vi "ClimbWeightQueue.vi"(7 "Action":T1, 8 "error in (no error)":errorcluster, 9 "Swing Out?":bool, 10 "ClimbWeightSol4":T2={"DevStatus"={"status"=FALSE, "code"=0, "source"=""}, "Solenoid Module"=enum."Solenoid Module 1", "Forward Solenoid Channel"=enum."Invalid", "Reverse Solenoid Channel"=enum."Invalid"}, 11 "ClimbWeightSol3":T2={"DevStatus"={"status"=FALSE, "code"=0, "source"=""}, "Solenoid Module"=enum."Solenoid Module 1", "Forward Solenoid Channel"=enum."Invalid", "Reverse Solenoid Channel"=enum."Invalid"}) -> (0 "error out":errorcluster)   [LabVIEW 2013]
uses:
  <vilib>/Rock Robotics/WPI/Solenoid/WPI_SolenoidDevRef.ctl
  <vilib>/Rock Robotics/SystemInterfaces/Typedef/FPGA_TypedefSolenoidModule.ctl
  <vilib>/Rock Robotics/WPI/Solenoid/WPI_SolenoidChannel.ctl
  ActionEnum.ctl
  <vilib>/Rock Robotics/WPI/Solenoid/WPI_SolenoidValue.ctl
  <vilib>/Rock Robotics/WPI/Solenoid/WPI_SolenoidSetEnum.vi
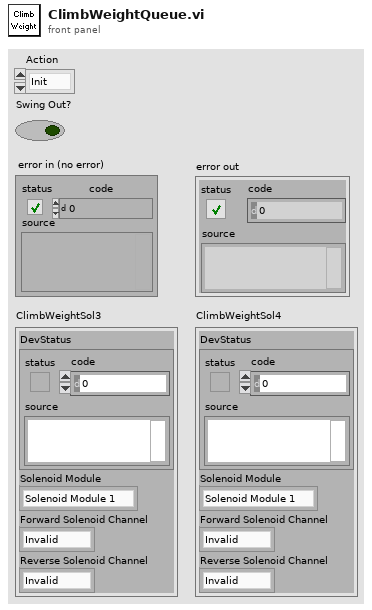
[diagram p1: front panel]
types:
  T1 = typedef "ActionEnum.ctl" = enum16{"Init", "SetValue"}
  T2 = typedef "WPI_SolenoidDevRef.ctl" = cluster{"DevStatus":errorcluster, "Solenoid Module":T3, "Forward Solenoid Channel":T4, "Reverse Solenoid Channel":T4}
  T3 = typedef "FPGA_TypedefSolenoidModule.ctl" = enum16{"Solenoid Module 1", "Solenoid Module 2"}
  T4 = typedef "WPI_SolenoidChannel.ctl" = enum8{"Solenoid 1", "Solenoid 2", "Solenoid 3", "Solenoid 4", "Solenoid 5", "Solenoid 6", "Solenoid 7", "Solenoid 8", "Invalid"}
  T5 = typedef "WPI_SolenoidValue.ctl" = enum16{"Off", "On", "Forward", "Reverse"}
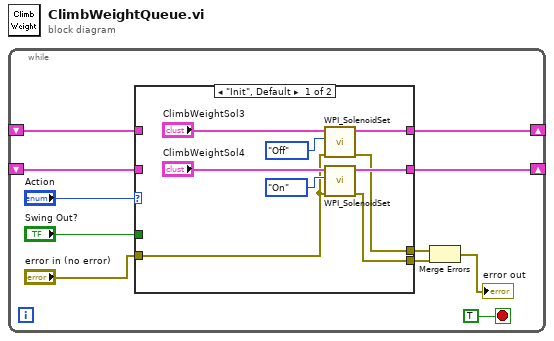
[diagram p0: block diagram]
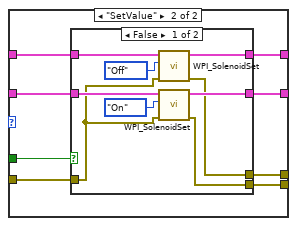
[diagram p2: hidden frame]
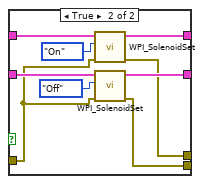
[diagram p3: hidden frame]
diagram:
  n1 = while {
    shift-right: [w6] -> _
    shift-left: _ -> [w10]
    shift-right: [w7] -> _
    shift-left: _ -> [w9]
    stop <- TRUE stop-if-true
    n2 = case shown="\"Init\", Default" "Action" {
      tunnel: [w17 w28] -> w6
      tunnel: [w15 w27] -> w7
      tunnel: w10 -> [_ w24]
      tunnel: w9 -> [_ w23]
      tunnel: "Swing Out?" -> [_ w26]
      tunnel: "error in (no error)" -> [w14 w25]
      tunnel: [w13 w22] -> w3
      tunnel: [w12 w21] -> w2
      frame "Init", Default {
        n3 = call-poly <vilib>:"WPI_SolenoidSet.vi"("error in (no error)"=w14, "Value"=WPI_SolenoidValue."Off", "SolenoidDevRef"="ClimbWeightSol3") -> ("error out"=w13:errorcluster, "SolenoidDevRef"=w17:T2)  [unwired: 7 in]
        n4 = call-poly <vilib>:"WPI_SolenoidSet.vi"("error in (no error)"=w14, "Value"=WPI_SolenoidValue."On", "SolenoidDevRef"="ClimbWeightSol4") -> ("error out"=w12:errorcluster, "SolenoidDevRef"=w15:T2)  [unwired: 7 in]
      }
      frame "SetValue" {
        n5 = case shown="False" w26 {
          tunnel: [w34 w45] -> w27
          tunnel: [w35 w46] -> w28
          tunnel: w25 -> [w31 w40]
          tunnel: w24 -> [w33 w42]
          tunnel: w23 -> [w32 w41]
          tunnel: [w29 w39] -> w21
          tunnel: [w30 w38] -> w22
          frame False {
            n6 = call-poly <vilib>:"WPI_SolenoidSet.vi"("error in (no error)"=w31, "Value"=WPI_SolenoidValue."Off", "SolenoidDevRef"=w33) -> ("error out"=w30:errorcluster, "SolenoidDevRef"=w35:T2)  [unwired: 7 in]
            n7 = call-poly <vilib>:"WPI_SolenoidSet.vi"("error in (no error)"=w31, "Value"=WPI_SolenoidValue."On", "SolenoidDevRef"=w32) -> ("error out"=w29:errorcluster, "SolenoidDevRef"=w34:T2)  [unwired: 7 in]
          }
          frame True {
            n8 = call-poly <vilib>:"WPI_SolenoidSet.vi"("error in (no error)"=w40, "Value"=WPI_SolenoidValue."On", "SolenoidDevRef"=w42) -> ("error out"=w38:errorcluster, "SolenoidDevRef"=w46:T2)  [unwired: 7 in]
            n9 = call-poly <vilib>:"WPI_SolenoidSet.vi"("error in (no error)"=w40, "Value"=WPI_SolenoidValue."Off", "SolenoidDevRef"=w41) -> ("error out"=w39:errorcluster, "SolenoidDevRef"=w45:T2)  [unwired: 7 in]
          }
        }
      }
    }
    n10 = Merge Errors(w3, w2) -> (→"error out":errorcluster)
  }
